vi "Command Hybrid Turn to Heading.vi"(7 "Startup":bool, 8 "Timeout":dbl=5.0, 9 "Translation (Throttle)":dbl=0.4, 11 "Heading":dbl=155.0) -> (2 "Right Wheel":dbl, 3 "Left Wheel":dbl, 4 "Reinit":bool, 6 "Completed":bool=TRUE)   [LabVIEW 2017]
uses:
  Utility VIs/Refnum Names.vi
  Drive/Drive Globals.vi
panel:
  out "Current Error":dbl=-0.3466796875
  out "Outputs":T1(graph)={"Current Error"=-0.3466796875, "Left Out"=-16.9974, "Right Out"=16.9974, "y"=0.0}
  in  "Ki":dbl=0.08
  in  "Kp":dbl=0.018
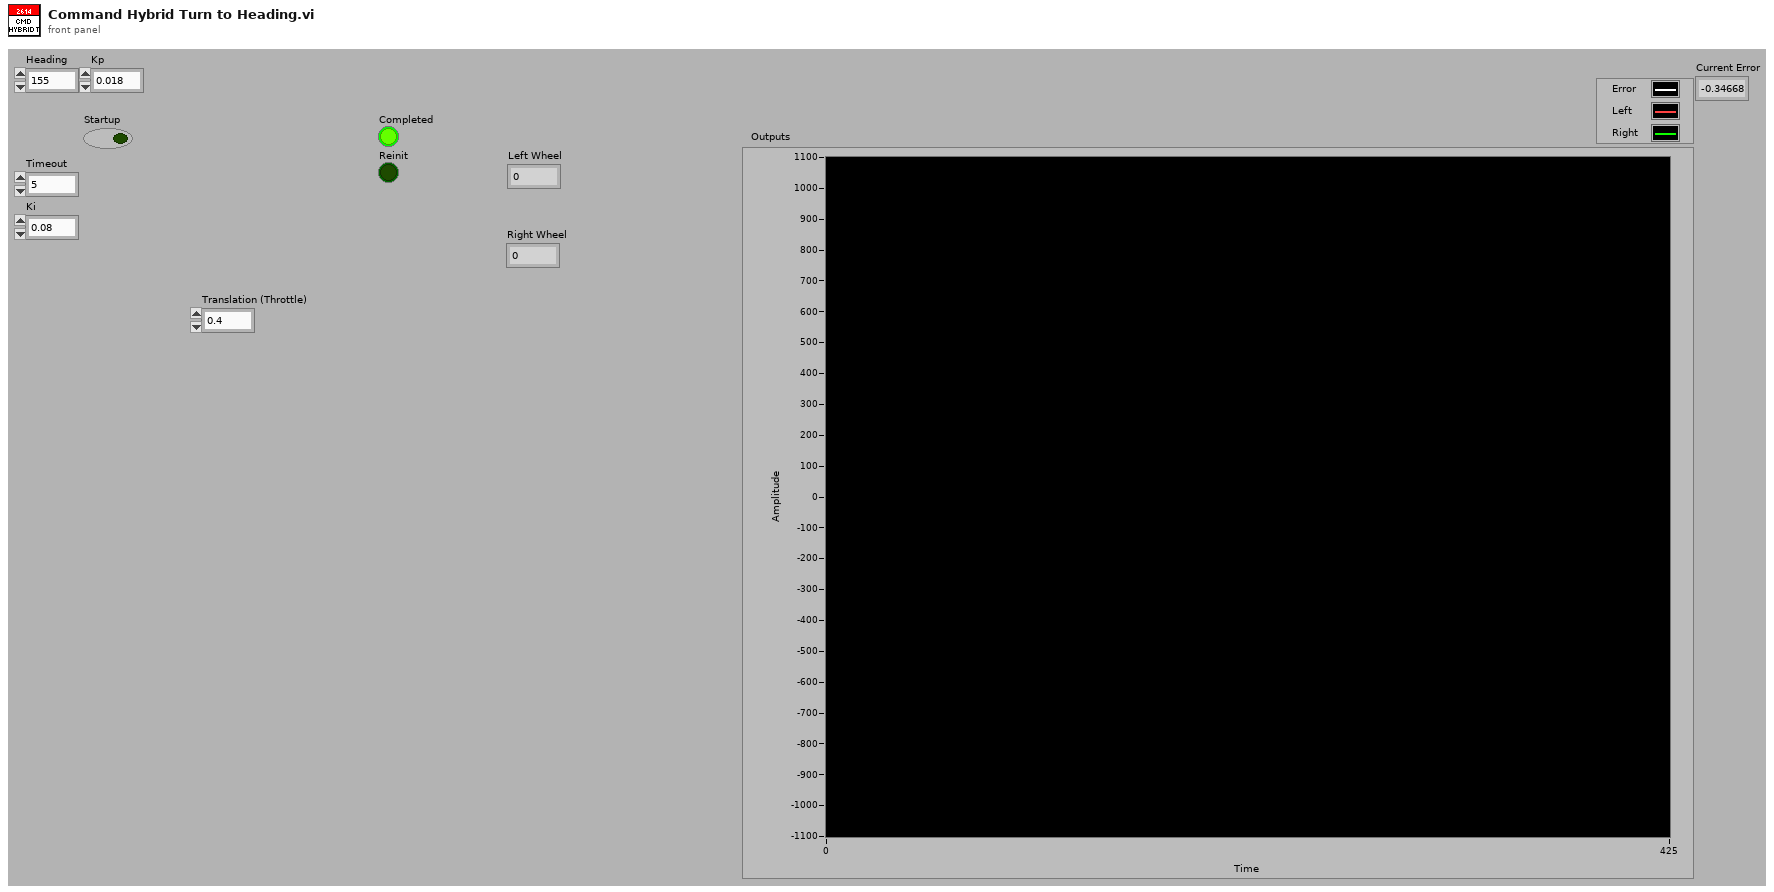
[diagram p1: front panel]
types:
  T1 = cluster{"Current Error":dbl, "Left Out":dbl, "Right Out":dbl, "y":dbl}
  T2 = typedef "CTRE_PigeonIMU_DeviceRef.ctl" = cluster{"DeviceStatus":errorcluster, "Device Number":u8, "Type":T3, "Device ID":u32, "Handle":u64, "UsageFrame":u32, "Library Path":path}
  T3 = typedef "CTRE_PigeonIMU_ConnectionType.ctl" = u32
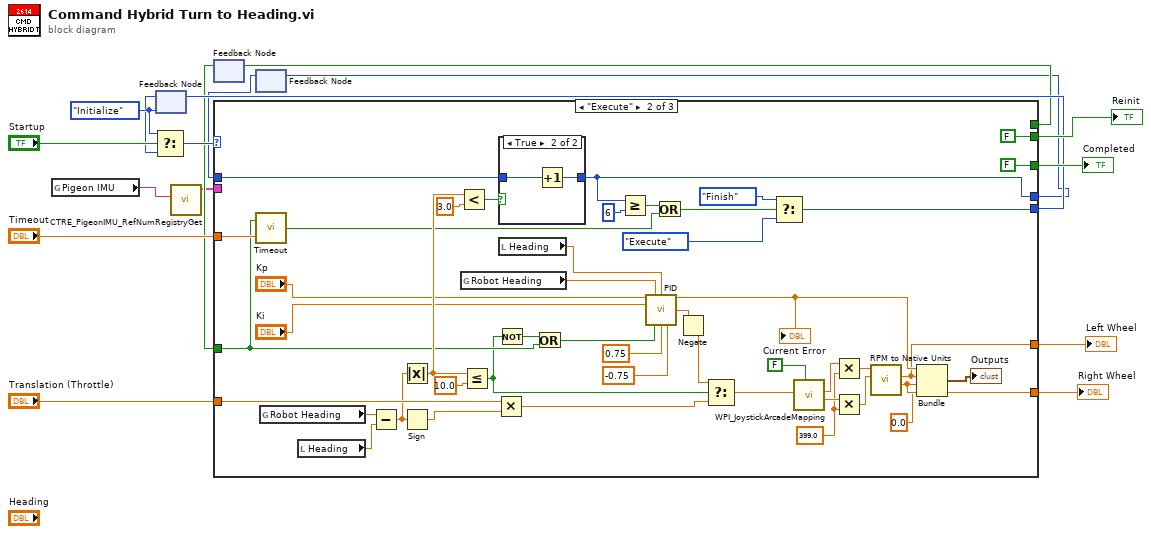
[diagram p0: block diagram]
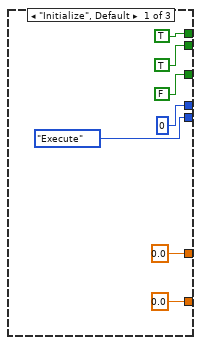
[diagram p2: hidden frame]
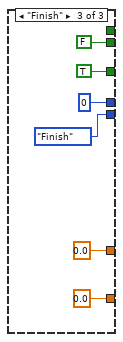
[diagram p4: hidden frame]
diagram:
  w15 = enum16{"Initialize", "Execute", "Finish"}."Initialize"
  n1 = global read "Refnum Names.vi" "Pigeon IMU"() -> (w2:string)
  n2 = feedback #1(w15) -> (w11:enum16{"Initialize", "Execute", "Finish"})
  n3 = Select(t=w15, s="Startup", f=w11) -> (s? t:f=w16:enum16{"Initialize", "Execute", "Finish"})
  n4 = call <vilib>:"CTRE_PigeonIMU_RefNumRegistryGet.vi"("refnum name"=w2) -> ("PigeonIMUDevRef"=w1:T2)  [unwired: 9 in, 1 out]
  n5 = feedback #2() -> (w5:bool)  [unwired: 1 in]
  n6 = feedback #3() -> (w3:i32)  [unwired: 1 in]
  n7 = case shown="\"Execute\"" w16 {
    tunnel: [FALSE FALSE TRUE] -> w14
    tunnel: [TRUE FALSE FALSE] -> w13
    tunnel: [enum16{"Initialize", "Execute", "Finish"}."Execute" w66 enum16{"Initialize", "Execute", "Finish"}."Finish"] -> w12
    tunnel: [0.0 ("Left Wheel Velocity") w34 0.0] -> w10
    tunnel: [0.0 ("Right Wheel Velocity") w33 0.0] -> w9
    tunnel: "Translation (Throttle)" -> [_ w54 _]
    tunnel: "Timeout" -> [_ w48 _]
    tunnel: w5 -> [_ w45 _]
    tunnel: [TRUE _ _] -> w6
    tunnel: w3 -> [_ w44 _]
    tunnel: [0 w42 0] -> w4
    tunnel: w1 -> [_ _ _]
    frame "Initialize", Default {
    }
    frame "Execute" {
      w63 = 399.0 ("y")
      n8 = call "Timeout.vi"("Timeout"=w48, "Initialize"=w45) -> ("Timed Out?"=w46:bool)
      n9 = global read "Drive Globals.vi" "Robot Heading"() -> (w60:dbl)
      n10 = local read "Heading"() -> (w59:dbl)
      n11 = Subtract(x=w60, y=w59) -> (x-y=w29:dbl)
      n12 = Absolute Value(x=w29) -> (abs(x)=w56:dbl)
      n13 = Sign(1:w29) -> (0:w30:dbl)
      n14 = Less?(x=w56, y=3.0) -> (x < y?=w43:bool)
      n15 = global read "Drive Globals.vi" "Robot Heading"() -> (w51:dbl)
      n16 = Less Or Equal?(x=w56, y=10.0) -> (x <= y?=w28:bool)
      n17 = Multiply(x=w54, y=w30) -> (x*y=w31:dbl)
      n18 = Not(x=w28) -> (.not. x?=w27:bool)
      n19 = case shown="True" w43 {
        tunnel: w44 -> [w71 w73]
        tunnel: [w71 w72] -> w42
        frame False {
        }
        frame True {
          n20 = Increment(x=w73) -> (x+1=w72:i32)
        }
      }
      n21 = local read "Heading"() -> (w50:dbl)
      n22 = Or(x=w27, y=w45) -> (x .or. y?=w32:bool)
      n23 = Greater Or Equal?(x=w42, y=6) -> (x >= y?=w40:bool)
      n24 = call "PID.vi"("Kp"="Kp", "Process Variable"=w51, "Goal"=w50, "Ki"="Ki", "Reinit"=w32, "Max Ouput"=0.75, "Min Output"=-0.75) -> ("Current Error"=w36:dbl, "Command"=w53:dbl)  [unwired: 6 in, 1 out]
      "Current Error" <- w36
      n25 = Or(x=w40, y=w46) -> (x .or. y?=w47:bool)
      n26 = Negate(x=w53) -> (-x=w25:dbl)
      n27 = Select(t=w25, s=w28, f=w31) -> (s? t:f=w52:dbl)
      n28 = Select(t=enum16{"Initialize", "Execute", "Finish"}."Finish", s=w47, f=enum16{"Initialize", "Execute", "Finish"}."Execute") -> (s? t:f=w66:enum16{"Initialize", "Execute", "Finish"})
      n29 = call <vilib>:"WPI_JoystickArcadeMapping.vi"("Square Inputs"=FALSE, "X axis value"=w52) -> ("Right Motor Value"=w64:dbl, "Left Motor Value"=w65:dbl)  [unwired: 8 in]
      n30 = Multiply(x=w65, y=w63) -> (x*y=w62:dbl)
      n31 = Multiply(x=w64, y=w63) -> (x*y=w61:dbl)
      n32 = call "RPM to Native Units.vi"("Right RPM"=w61, "Left RPM"=w62) -> ("Right Out"=w33:dbl, "Left Out"=w34:dbl)  [unwired: 6 in, 1 out]
      n33 = Bundle("Current Error"=w36, "Left Out"=w34, "Right Out"=w33, "y"=0.0) -> (→"Outputs":T1)  [unwired: 1 in]
    }
    frame "Finish" {
    }
  }
  "Completed" <- w14
  "Reinit" <- w13
  "Left Wheel" <- w10
  "Right Wheel" <- w9
  n34 = feedback-in #1(w12) -> ()
  n35 = feedback-in #2(w6) -> ()
  n36 = feedback-in #3(w4) -> ()
